vi "init.vi"(0 "Constant Analog Output Voltage Test in":refnum<class "Current Linear Test.lvclass">, 1 "DAQ Channel 1":refnum<k21>, 2 "ConfigureILCStrategy":refnum<class "IConfigureILCStrategy.lvclass">, 3 "Counts Per Iteration":i32, 4 "Samples To Average":i32, 5 "error in (no error)":errorcluster, 6 "DAQ Channel 2":refnum<k21>, 7 "Log":refnum<class "ITestLog.lvclass">, 8 "Test Scenario":T1, 9 "Resistance":dbl format="%.3f", 10 "Signal Name":string) -> (14 "Constant Analog Output Voltage Test  out":refnum<class "Current Linear Test.lvclass">, 19 "error out":errorcluster)   [LabVIEW 2015, in "Current Linear Test.lvclass"]
uses:
  Current Linear Test.lvclass
  Model/TestLog/ITestLog/ITestLog.lvclass
  Typedefs/TestScenarioTypes.ctl
  Model/ConfigureILCStrategy/IConfigureILCStrategy/IConfigureILCStrategy.lvclass
  Current Linear Test.lvclass/Current Linear Test.ctl
  Typedefs/ILCBTTypedefs.lvlib
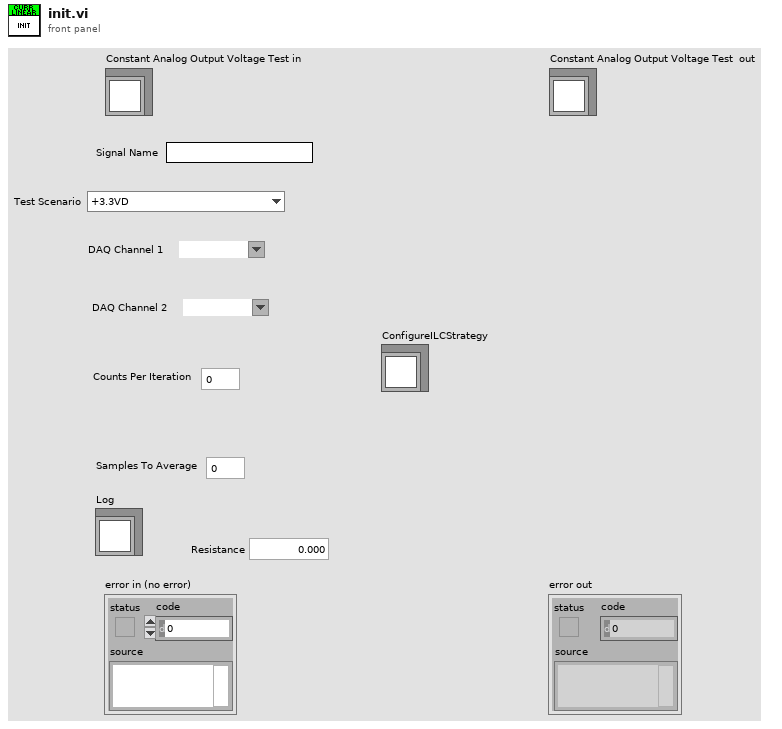
[diagram p1: front panel]
types:
  T1 = typedef "ILCBTTypedefs.lvlib/TestScenarioTypes.ctl" = enum16{"+3.3VD", "+5.1V", "+24V", "RELVALV1", "RELVALV2", "Verify DAC_A = -1.00A", "Verify DAC_A = -0.75A", "Verify DAC_A = -0.50A", "Verify DAC_A = -0.25A", "Verify DAC_A = 0.00A", "Verify DAC_A = 0.25A", "Verify DAC_A = 0.50A", "Verify DAC_A = 0.75A", "Verify DAC_A = 1.00A", "Verify DAC_B = -1.00A", "Verify DAC_B = -0.75A", "Verify DAC_B = -0.50A", "Verify DAC_B = -0.25A", "Verify DAC_B = 0.00A", "Verify DAC_B = 0.25A", "Verify DAC_B = 0.50A", "Verify DAC_B = 0.75A", "Verify DAC_B = 1.00A", "Set DAC_A = -1.00A", "Set DAC_A = -0.75A", "Set DAC_A = -0.50A", "Set DAC_A = -0.25A", "Set DAC_A = 0.00A", "Set DAC_A = 0.25A", "Set DAC_A = 0.50A", "Set DAC_A = 0.75A", "Set DAC_A = 1.00A", "Set DAC_B = -1.00A", "Set DAC_B = -0.75A", "Set DAC_B = -0.50A", "Set DAC_B = -0.25A", "Set DAC_B = 0.00A", "Set DAC_B = 0.25A", "Set DAC_B = 0.50A", "Set DAC_B = 0.75A", "Set DAC_B = 1.00A", "Set MTR_PWR = On", "Set MTR_PWR = Off", "Set OUTPUT = On", "Set OUTPUT = Off", "Verify OUTPUT = On", "Verify OUTPUT = Off", "Verify POWER = Ok", "Verify POWER = Fail", "Verify AMP1 = Ok", "Verify AMP1 = Fail", "Verify AMP2 = Ok", "Verify AMP2 = Fail", "P1 0%", "P1 25%", "P1 50%", "P1 75%", "P1 100%", "P2 0%", "P2 25%", "P2 50%", "P2 75%", "P2 100%", "P3 0%", "P3 25%", "P3 50%", "P3 75%", "P3 100%", "P4 0%", "P4 25%", "P4 50%", "P4 75%", "P4 100%", "DCA 1 Linearity", "DCA 2 Linearity"}
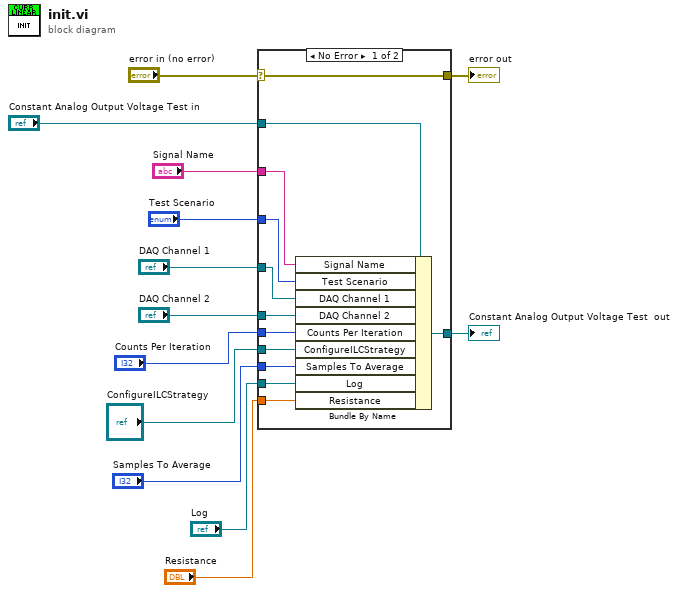
[diagram p0: block diagram]
diagram:
  n1 = case shown="No Error" "error in (no error)" {
    selector: "error in (no error)" -> [w25 w27]
    tunnel: [w25 w27] -> w12
    tunnel: [w23 w26] -> w10
    tunnel: "Constant Analog Output Voltage Test in" -> [w24 w26]
    tunnel: "DAQ Channel 1" -> [w18 _]
    tunnel: "Samples To Average" -> [w22 _]
    tunnel: "Log" -> [w21 _]
    tunnel: "Signal Name" -> [w20 _]
    tunnel: "Test Scenario" -> [w19 _]
    tunnel: "DAQ Channel 2" -> [w17 _]
    tunnel: "Resistance" -> [w16 _]
    tunnel: "Counts Per Iteration" -> [w15 _]
    tunnel: "ConfigureILCStrategy" -> [w14 _]
    frame No Error {
      n2 = Bundle By Name(cluster=w24, "Signal Name"=w20, "Test Scenario"=w19, "DAQ Channel 1"=w18, "DAQ Channel 2"=w17, "Counts Per Iteration"=w15, "ConfigureILCStrategy"=w14, "Samples To Average"=w22, "Log"=w21, "Resistance"=w16) -> (w23:refnum<class "Current Linear Test.lvclass">)
    }
    frame Error {
    }
  }
  "error out" <- w12
  "Constant Analog Output Voltage Test  out" <- w10
